vi "Event Handler - Variables View - Key Down.vi"(4 "User Parameter":T1, 5 "Event Data":cluster{"keyCode":i16, "shift":i16}, 6 "Control Ref":refnum<k7>, 7 "Event Common Data":T2) -> (1 "Event Data Out":cluster{"keyCode":i16})   [LabVIEW 2021, in "Seq Edit Quick Drop.lvlib"]
uses:
  Seq Edit Quick Drop.lvlib
  Event Data.ctl
  Connection Type.ctl
  Event Response.ctl
  Message.ctl
  Command.ctl
  Key Codes Constants.vi
  Settings.vi
  <vilib>/Utility/SystemLogging/NI_SystemLogging.lvlib
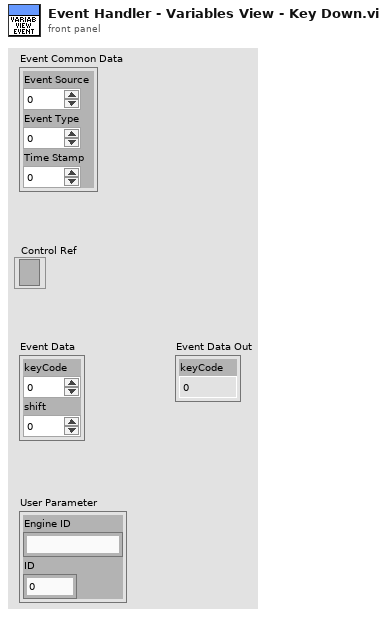
[diagram p1: front panel]
types:
  T1 = typedef "Seq Edit Quick Drop.lvlib/Event Data.ctl" = cluster{"Engine ID":string, "ID":i32}
  T2 = cluster{"Event Source":i32, "Event Type":u32, "Time Stamp":u32}
  T3 = typedef "Seq Edit Quick Drop.lvlib/Event Response.ctl" = cluster{"Connection Type":T4, "ID":i32}
  T4 = typedef "Seq Edit Quick Drop.lvlib/Connection Type.ctl" = enum16{"SequenceView", "SequenceList", "VariablesView"}
  T5 = cluster{"Key":string, "Modifiers":cluster{"SHIFT":bool, "CONTROL":bool, "ALT":bool}}
  T6 = cluster{"SHIFT":bool, "CONTROL":bool, "ALT":bool}
  T7 = typedef "Seq Edit Quick Drop.lvlib/Message.ctl" = cluster{"cmd":T8, "data":variant}
  T8 = typedef "Seq Edit Quick Drop.lvlib/Command.ctl" = enum16{"Init", "Get Application Manager", "Shortcut Activated", "Display Tools", "Tool Selected", "Timeout", "Error", "Close"}
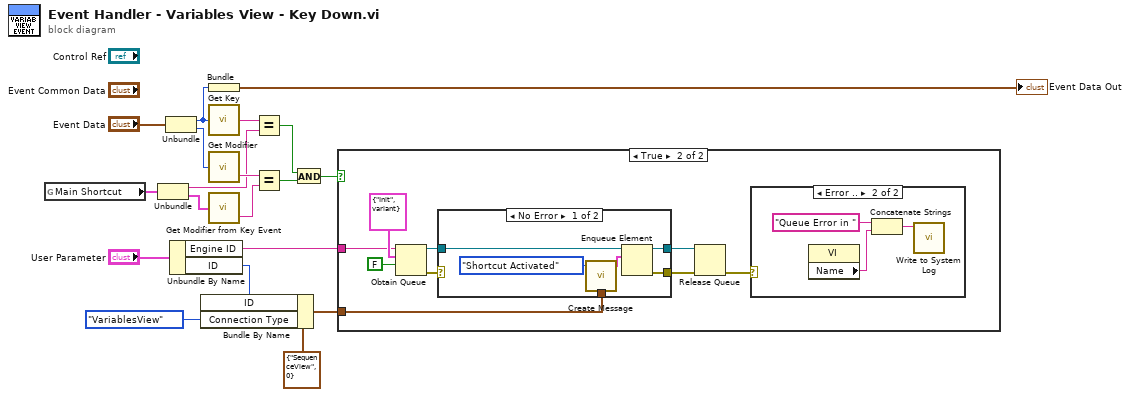
[diagram p0: block diagram]
diagram:
  n1 = global read "Settings.vi" "Main Shortcut"() -> (w13:T5)
  n2 = Unbundle(w13) -> ("Key"=w12:string, "Modifiers"=w2:T6)
  n3 = Unbundle("Event Data") -> ("keyCode"=w19:i16, "shift"=w18:i16)
  n4 = Unbundle By Name("User Parameter") -> ("Engine ID"=w10:string, "ID"=w7:i32)
  n5 = Bundle By Name(cluster=T3 {"Connection Type"=enum."SequenceView", "ID"=0} ("Event Response"), "ID"=w7, "Connection Type"=Connection_Type."VariablesView") -> (w6:T3)
  n6 = Bundle("keyCode"=w19) -> (→"Event Data Out":cluster{"keyCode":i16})  [unwired: 1 in]
  n7 = call "Get Key.vi"("Key Code"=w19) -> ("Key"=w17:string)
  n8 = call "Get Modifier.vi"("Modifier Code"=w18) -> ("Modifiers Concatenated"=w16:string)  [unwired: 1 out]
  n9 = call "Get Modifier from Key Event.vi"("Modifiers"=w2) -> ("Modifiers Concatenated"=w1:string)  [unwired: 1 out]
  n10 = Equal?(x=w17, y=w12) -> (x = y?=w15:bool)
  n11 = Equal?(x=w16, y=w1) -> (x = y?=w14:bool)
  n12 = And(x=w15, y=w14) -> (x .and. y?=w11:bool)
  n13 = case shown="True" w11 {
    tunnel: w10 -> [_ w24]
    tunnel: w6 -> [_ w22]
    frame False {
    }
    frame True {
      n14 = Obtain Queue(name (unnamed)=w24, element data type=T7 {"cmd"=enum."Init", "data"=variant} ("msg"), create if not found? (T)=FALSE) -> (queue out=w26:refnum<queue>, error out=w25:errorcluster)  [unwired: 2 in, 1 out]
      n15 = case shown="No Error" w25 {
        selector: w25 -> [_ w39]
        tunnel: w26 -> [w35 w38]
        tunnel: [w34 w39] -> w23
        tunnel: w22 -> [w33 _]
        tunnel: [w32 w38] -> w20
        frame No Error {
          n16 = call "Create Message.vi"("cmd"=Command."Shortcut Activated", "data"=w33) -> ("msg"=w36:T7)  [unwired: 2 in]
          n17 = Enqueue Element(queue=w35, element=w36) -> (queue out=w32:refnum<queue>, error out=w34:errorcluster)  [unwired: 2 in, 1 out]
        }
        frame Error {
        }
      }
      n18 = Release Queue(queue=w20, error in (no error)=w23) -> (error out=w21:errorcluster)  [unwired: 1 in, 2 out]
      n19 = case shown="Error .." w21 {
        frame No Error {
        }
        frame Error {
          n20 = property class="VI"() -> ("Name"=w30:string)  [unwired: 2 in, 2 out]
          n21 = Concatenate Strings("Queue Error in " ("string"), w30) -> (w29:string)
          n22 = call <vilib>:"Write to System Log.vi"("message"=w29) -> ()  [unwired: 10 in, 1 out]
        }
      }
    }
  }
